vi "采集切换.vi"(10 "工位":enum16{"工位一", "工位二"}(ring), 11 "采集方式":enum16{"板卡采集", "PGI采集"}(ring)) -> ()   [LabVIEW 2020]
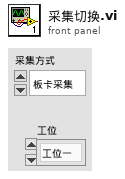
[diagram p1: front panel]
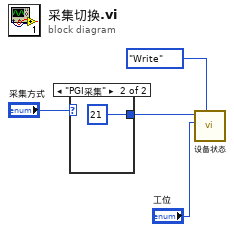
[diagram p0: block diagram]
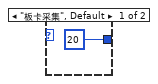
[diagram p2: hidden frame]
diagram:
  n1 = case shown="\"PGI采集\"" "采集方式" {
    tunnel: [i16 20 ("Status_Write") i16 21 ("Status_Write")] -> w1
    frame "板卡采集", Default {
    }
    frame "PGI采集" {
    }
  }
  n2 = call "设备状态.vi"("枚举"=enum16{"Read", "Write"}."Write", "工位"="工位", "Status_Write"=w1) -> ()  [unwired: 8 in, 1 out]
